vi "GOOP4_Sub_Create.vi"(8 "error in (no error)":errorcluster, 9 "Str":string, 10 "i":i32, 11 "reference in":refnum<class "GOOP4_Sub.lvclass">) -> (0 "error out":errorcluster, 3 "reference out":refnum<class "GOOP4_Sub.lvclass">)   [LabVIEW 2019, in "GOOP4_Sub.lvclass"]
uses:
  GOOP4_Sub.lvclass
  C:/Users/Tiba/Desktop/GOOP4_CreateObjects_Open_GDS/GOOP4_Base_class/GOOP4_Base.lvclass
  GOOP4_Base_class/GOOP4_Base.lvclass
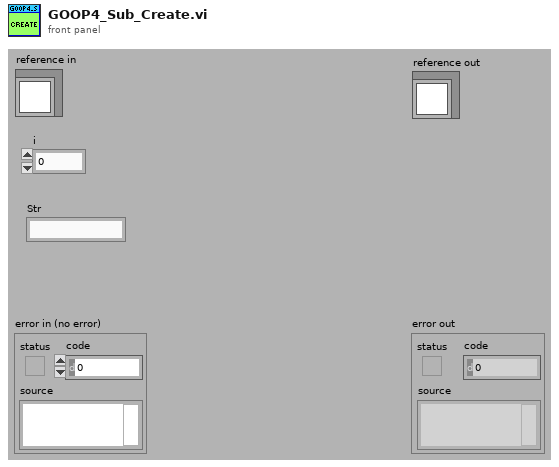
[diagram p1: front panel]
types:
  T1 = typedef "GOOP4_Sub.lvclass/ObjectAttributes.ctl" = cluster{"Str":string, "Boolean":bool}
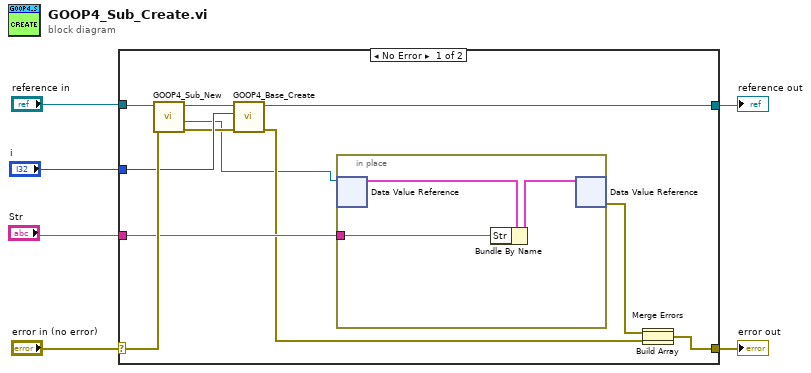
[diagram p0: block diagram]
diagram:
  n1 = case shown="No Error" "error in (no error)" {
    selector: "error in (no error)" -> [w17 w23]
    tunnel: [w15 w23] -> w5
    tunnel: "reference in" -> [w18 w22]
    tunnel: [w10 w22] -> w4
    tunnel: "i" -> [w14 _]
    tunnel: "Str" -> [w13 _]
    frame No Error {
      n2 = call "GOOP4_Sub_New.vi"("error in (no error)"=w17, "reference in"=w18) -> ("error out"=w9:errorcluster, "DVRRefOut"=w7:refnum<data-value>, "reference out"=w11:refnum<class "GOOP4_Sub.lvclass">)  [unwired: 6 in, 1 out]
      n3 = call "GOOP4_Base_Create.vi"("error in (no error)"=w9, "i"=w14, "reference in"=w11) -> ("error out"=w8:errorcluster, "reference out"=w10:refnum<class "GOOP4_Sub.lvclass">)  [unwired: 7 in]
      n4 = in-place {
        in-place-border: w13 -> [w19]
        n5 = in-place-dvr #1(w7) -> (w20:T1)  [unwired: 1 out]
        n6 = Bundle By Name(cluster=w20, "Str"=w19) -> (w21:T1)
        n7 = in-place-dvr #1(w21) -> (w16:errorcluster)  [unwired: 1 out]
      }
      n8 = Build Array(w16, w8) -> (w12:errorcluster[])
      n9 = Merge Errors(w12) -> (w15:errorcluster)
    }
    frame Error {
    }
  }
  "error out" <- w5
  "reference out" <- w4
